vi "Insert Start Message.vi"(8 "error in (no error)":errorcluster, 10 "Start Time":timestamp, 11 "AODAcq in":refnum<class "AODAcq.lvclass">) -> (0 "error out":errorcluster, 3 "AODAcq out":refnum<class "AODAcq.lvclass">)   [LabVIEW 2011, in "AODAcq.lvclass"]
uses:
  AODAcq.lvclass
  <vilib>/Utility/error.llb/DialogType.ctl
  AcquistionObject/AcquistionObject.lvclass
  Database/SessionPrimary.ctl
  Database/AodScanPrimary.ctl
  <vilib>/addons/database/NI_Database_API.lvlib
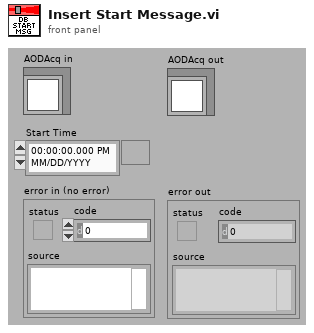
[diagram p1: front panel]
types:
  T1 = typedef "DialogType.ctl" = u16
  T2 = cluster{"setup":u8, "subject_id":i32, "session_start_time":dbl, "aod_scan_start_time":dbl, "aod_scan_filename":string, "x_coordinate":dbl, "y_coordinate":dbl, "z_coordinate":dbl, "objective":string, "motion_planes":u8, "pmt_green":dbl, "pmt_red":dbl, "preamplifier_green":string, "preamplifier_red":string, "attenuator_degrees":dbl, "scan_power":dbl, "depth":dbl, "gdd":dbl}
  T3 = cluster{"setup":u8, "subject_id":i32, "session_start_time":dbl, "aod_volume_start_time":dbl, "aod_volume_filename":string, "x_coordinate":dbl, "y_coordinate":dbl, "z_coordinate":dbl, "objective":string, "x_range":dbl, "y_range":dbl, "z_range":dbl, "x_resolution":dbl, "y_resolution":dbl, "z_resolution":dbl, "pmt_green":dbl, "pmt_red":dbl, "preamplifier_green":string, "preamplifier_red":string, "attenuator_degrees":dbl, "scan_power":dbl, "depth":dbl, "gdd":dbl, "reps":dbl}
  T4 = typedef "NI_Database_API.lvlib/Conn ObjectReference.ctl" = refnum<k1>
  T5 = typedef "SessionPrimary.ctl" = cluster{"setup":u8, "subject_id":i32, "session_start_time":dbl}
  T6 = typedef "AodScanPrimary.ctl" = cluster{"setup":u8, "subject_id":i32, "session_start_time":dbl, "aod_scan_start_time":dbl}
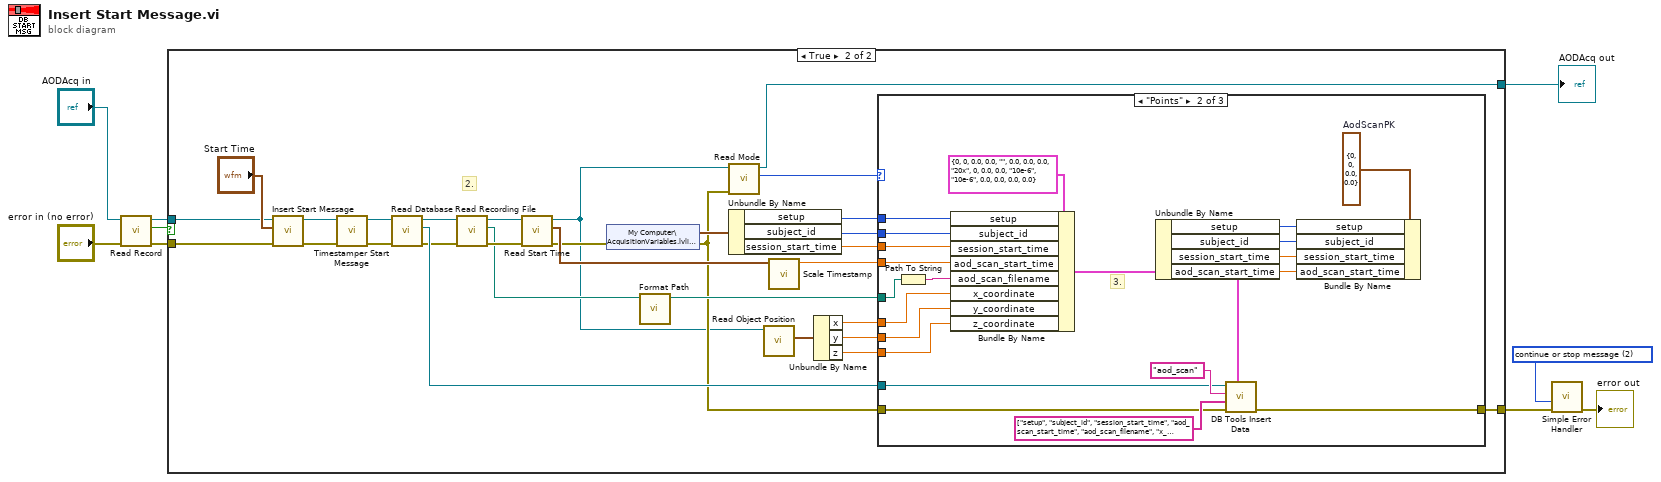
[diagram p0: block diagram]
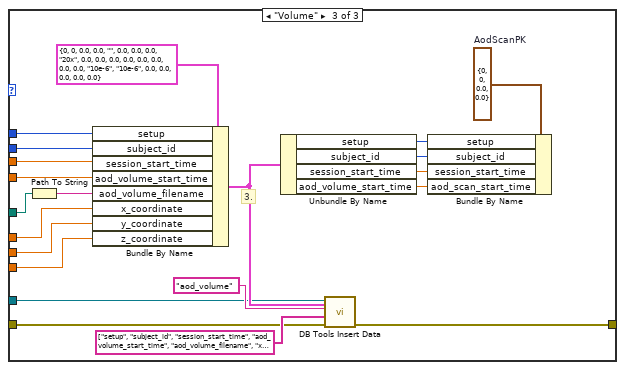
[diagram p4: hidden frame]
diagram:
  w2 = T1 2 items=["no dialog", "OK message", "continue or stop message", "OK message + warnings", "continue/stop + warnings"] ("type of dialog (OK msg:1)")
  n1 = call-dynamic "Read Record.vi"("error in (no error)"="error in (no error)", "AODAcq in"="AODAcq in") -> ("error out"=w7:errorcluster, "Record"=w5:bool, "AODAcq out"=w6:refnum<class "AODAcq.lvclass">)  [unwired: 7 in]
  n2 = case shown="True" w5 {
    tunnel: [w11 w24] -> w3
    tunnel: w7 -> [w11 w19]
    tunnel: w6 -> [w10 w17]
    tunnel: [w10 w18] -> w4
    frame False {
    }
    frame True {
      # "2."
      n3 = call-parent "Insert Start Message.vi"("error in (no error)"=w19, "Start Time"="Start Time", "AcquistionObject in"=w17) -> ("error out"=w23:errorcluster, "AcquistionObject out"=w21:refnum<class "AODAcq.lvclass">)  [unwired: 7 in]
      n4 = call-dynamic "Timestamper Start Message.vi"("error in (no error)"=w23, "AcquistionObject in"=w21) -> ("error out"=w22:errorcluster, "AcquistionObject out"=w20:refnum<class "AODAcq.lvclass">)  [unwired: 8 in]
      n5 = call-dynamic "Read Database.vi"("error in (no error)"=w22, "AcquistionObject in"=w20) -> ("error out"=w35:errorcluster, "reference"=w36:T4, "AcquistionObject out"=w34:refnum<class "AODAcq.lvclass">)  [unwired: 7 in]
      n6 = call-dynamic "Read Recording File.vi"("error in (no error)"=w35, "AcquistionObject in"=w34) -> ("error out"=w37:errorcluster, "Recording File"=w31:path, "AcquistionObject out"=w38:refnum<class "AODAcq.lvclass">)  [unwired: 7 in]
      n7 = call-dynamic "Read Start Time.vi"("error in (no error)"=w37, "AcquistionObject in"=w38) -> ("error out"=w29:errorcluster, "Start Time"=w33:timestamp, "AcquistionObject out"=w15:refnum<class "AODAcq.lvclass">)  [unwired: 7 in]
      n8 = shared-variable "My Computer\\AcquisitionVariables.lvlib\\SessionPK"(error in=w29) -> (w28:T5, error out=w27:errorcluster)
      n9 = call "Format Path.vi"("Input path"=w31) -> ("Output path"=w30:path)  [unwired: 10 in]
      n10 = call-dynamic "Read Mode.vi"("error in (no error)"=w27, "AODAcq in"=w15) -> ("Mode"=w26:enum16{"Idle", "Points", "Volume"}, "AODAcq out"=w18:refnum<class "AODAcq.lvclass">)  [unwired: 7 in, 1 out]
      n11 = Unbundle By Name(w28) -> ("setup"=w40:u8, "subject_id"=w39:i32, "session_start_time"=w32:dbl)
      n12 = call-dynamic "Read Object Position.vi"("AODAcq in"=w15) -> ("Object Position"=w16:cluster{"x":dbl, "y":dbl, "z":dbl})  [unwired: 8 in, 2 out]
      n13 = call "Scale Timestamp.vi"("Time Stamp"=w33) -> ("Scaled timestamp"=w25:dbl)  [unwired: 10 in]
      n14 = Unbundle By Name(w16) -> ("x"=w14:dbl, "y"=w13:dbl, "z"=w12:dbl)
      n15 = case shown="\"Points\"" w26 {
        tunnel: w40 -> [_ w61 w82]
        tunnel: w39 -> [_ w60 w81]
        tunnel: w36 -> [_ w55 w76]
        tunnel: w32 -> [_ w53 w74]
        tunnel: w30 -> [_ w48 w70]
        tunnel: w27 -> [w42 w52 w73]
        tunnel: w25 -> [_ w51 w72]
        tunnel: [w42 w46 w68] -> w24
        tunnel: w14 -> [_ w45 w66]
        tunnel: w13 -> [_ w44 w65]
        tunnel: w12 -> [_ w43 w64]
        frame "Idle", Default {
        }
        frame "Points" {
          w49 = T6 {"setup"=0, "subject_id"=0, "session_start_time"=0.0, "aod_scan_start_time"=0.0}  # AodScanPK
          # "3."
          n16 = Path To String(path=w48) -> (string=w47:string)
          n17 = Bundle By Name(cluster=T2 {"setup"=0, "subject_id"=0, "session_start_time"=0.0, "aod_scan_start_time"=0.0, "aod_scan_filename"="", "x_coordinate"=0.0, "y_coordinate"=0.0, "z_coordinate"=0.0, "objective"="20x", "motion_planes"=0, "pmt_green"=0.0, "pmt_red"=0.0, "preamplifier_green"="10e-6", "preamplifier_red"="10e-6", "attenuator_degrees"=0.0, "scan_power"=0.0, "depth"=0.0, "gdd"=0.0} ("AodScanPK"), "setup"=w61, "subject_id"=w60, "session_start_time"=w53, "aod_scan_start_time"=w51, "aod_scan_filename"=w47, "x_coordinate"=w45, "y_coordinate"=w44, "z_coordinate"=w43) -> (w59:T2)
          n18 = Unbundle By Name(w59) -> ("setup"=w58:u8, "subject_id"=w57:i32, "session_start_time"=w56:dbl, "aod_scan_start_time"=w54:dbl)
          n19 = call <vilib>:"DB Tools Insert Data.vi"("data"=w59, "error in (no error)"=w52, "columns"=string[] ["setup", "subject_id", "session_start_time", "aod_scan_start_time", "aod_scan_filename", "x_coordinate", "y_coordinate", "z_coordinate", "objective", "motion_planes", "pmt_green", "pmt_red", "preamplifier_green", "preamplifier_red", "attenuator_degrees", "scan_power", "depth", "gdd"], "table"="aod_scan", "connection reference"=w55) -> ("error out"=w46:errorcluster)  [unwired: 5 in, 1 out]
          n20 = Bundle By Name(cluster=w49, "setup"=w58, "subject_id"=w57, "session_start_time"=w56, "aod_scan_start_time"=w54) -> ()  [unwired: 1 out]
        }
        frame "Volume" {
          w71 = T6 {"setup"=0, "subject_id"=0, "session_start_time"=0.0, "aod_scan_start_time"=0.0}  # AodScanPK
          # "3."
          n21 = Path To String(path=w70) -> (string=w69:string)
          n22 = Bundle By Name(cluster=T3 {"setup"=0, "subject_id"=0, "session_start_time"=0.0, "aod_volume_start_time"=0.0, "aod_volume_filename"="", "x_coordinate"=0.0, "y_coordinate"=0.0, "z_coordinate"=0.0, "objective"="20x", "x_range"=0.0, "y_range"=0.0, "z_range"=0.0, "x_resolution"=0.0, "y_resolution"=0.0, "z_resolution"=0.0, "pmt_green"=0.0, "pmt_red"=0.0, "preamplifier_green"="10e-6", "preamplifier_red"="10e-6", "attenuator_degrees"=0.0, "scan_power"=0.0, "depth"=0.0, "gdd"=0.0, "reps"=0.0} ("AodScanPK"), "setup"=w82, "subject_id"=w81, "session_start_time"=w74, "aod_volume_start_time"=w72, "aod_volume_filename"=w69, "x_coordinate"=w66, "y_coordinate"=w65, "z_coordinate"=w64) -> (w80:T3)
          n23 = Unbundle By Name(w80) -> ("setup"=w79:u8, "subject_id"=w78:i32, "session_start_time"=w77:dbl, "aod_volume_start_time"=w75:dbl)
          n24 = call <vilib>:"DB Tools Insert Data.vi"("data"=w80, "error in (no error)"=w73, "columns"=string[] ["setup", "subject_id", "session_start_time", "aod_volume_start_time", "aod_volume_filename", "x_coordinate", "y_coordinate", "z_coordinate", "objective", "x_range", "y_range", "z_range", "x_resolution", "y_resolution", "z_resolution", "pmt_green", "pmt_red", "preamplifier_green", "preamplifier_red", "attenuator_degrees", "scan_power", "depth", "gdd", "reps"], "table"="aod_volume", "connection reference"=w76) -> ("error out"=w68:errorcluster)  [unwired: 5 in, 1 out]
          n25 = Bundle By Name(cluster=w71, "setup"=w79, "subject_id"=w78, "session_start_time"=w77, "aod_scan_start_time"=w75) -> ()  [unwired: 1 out]
        }
      }
    }
  }
  "AODAcq out" <- w4
  n26 = call <vilib>:"Simple Error Handler.vi"("type of dialog (OK msg:1)"=w2, "error in (no error)"=w3) -> ("error out"=→"error out":errorcluster)  [unwired: 3 in, 4 out]
